vi "SetClockParameters.vi"(7 "ClockEnable":bool, 8 "error in (no error)":errorcluster, 9 "DivideBy":u32=8, 10 "ClockSource":T1=1 items=["Internal Oscillator"=1, "External Trigger"=2, "Trigger & Oscillator"=3, "MasterSlave Bus"=4], 11 "BME_DG_G08 in":refnum<class "BME_DG_G08.lvclass">) -> (0 "error out":errorcluster, 3 "BME_DG_G08 out":refnum<class "BME_DG_G08.lvclass">)   [LabVIEW 2009]
uses:
  BME_DG_G08.lvclass
  LV-BME Interface/ClockSource.ctl
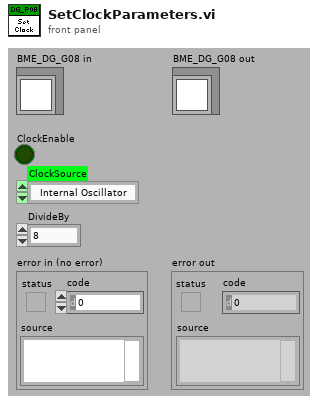
[diagram p1: front panel]
types:
  T1 = typedef "ClockSource.ctl" = i32
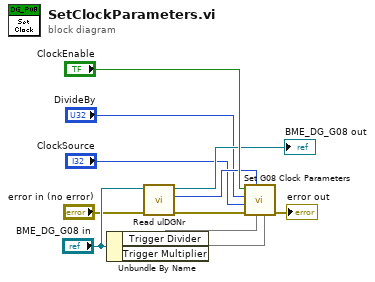
[diagram p0: block diagram]
diagram:
  n1 = Unbundle By Name("BME_DG_G08 in") -> ("Trigger Divider"=w2, "Trigger Multiplier"=w1)
  n2 = call-dynamic "Read ulDGNr.vi"("error in (no error)"="error in (no error)", "BME_DG_Base in"="BME_DG_G08 in") -> ("error out"=w7:errorcluster, "ulDGNr"=w6:u32, "BME_DG_Base out"=→"BME_DG_G08 out":refnum<class "BME_DG_G08.lvclass">)  [unwired: 6 in, 1 out]
  n3 = call "Set G08 Clock Parameters.vi"("Trigger Multiplier"=w1, "Trigger Divider"=w2, "DG Number"=w6, "error in (no error)"=w7, "Clock Source"="ClockSource", "Ocillator Divider"="DivideBy", "Clock Enable"="ClockEnable") -> ("error out"=→"error out":errorcluster)  [unwired: 4 in]
